vi "SortStates.vi"(0 "object in":refnum<class "StateReverse.lvclass">, 1 "StateTransitions":cluster{"StateTransitions":string[]}[](array[cluster]), 2 "CommentsTransitions":cluster{"StateTransitions":string[]}[](array[cluster]), 3 "StartState":string, 4 "ExitStates":string[](array[string]), 5 "error in (no error)":errorcluster, 8 "StateStrings":string[](array[string]), 9 "RemoveStatesNotInUse(True)":bool=TRUE) -> (14 "object out":refnum<class "StateReverse.lvclass">, 15 "States":T1[](array[typedef]), 19 "error out":errorcluster)   [LabVIEW 2016, in "StateReverse.lvclass"]
uses:
  <resource>/Framework/Providers/Open_GDS/UML/StateReverse_class/StateReverse.lvclass
  <resource>/Framework/Providers/Open_GDS/UML/ReversedEngineering/ReversedEngineering StateMachineStateInfo.ctl
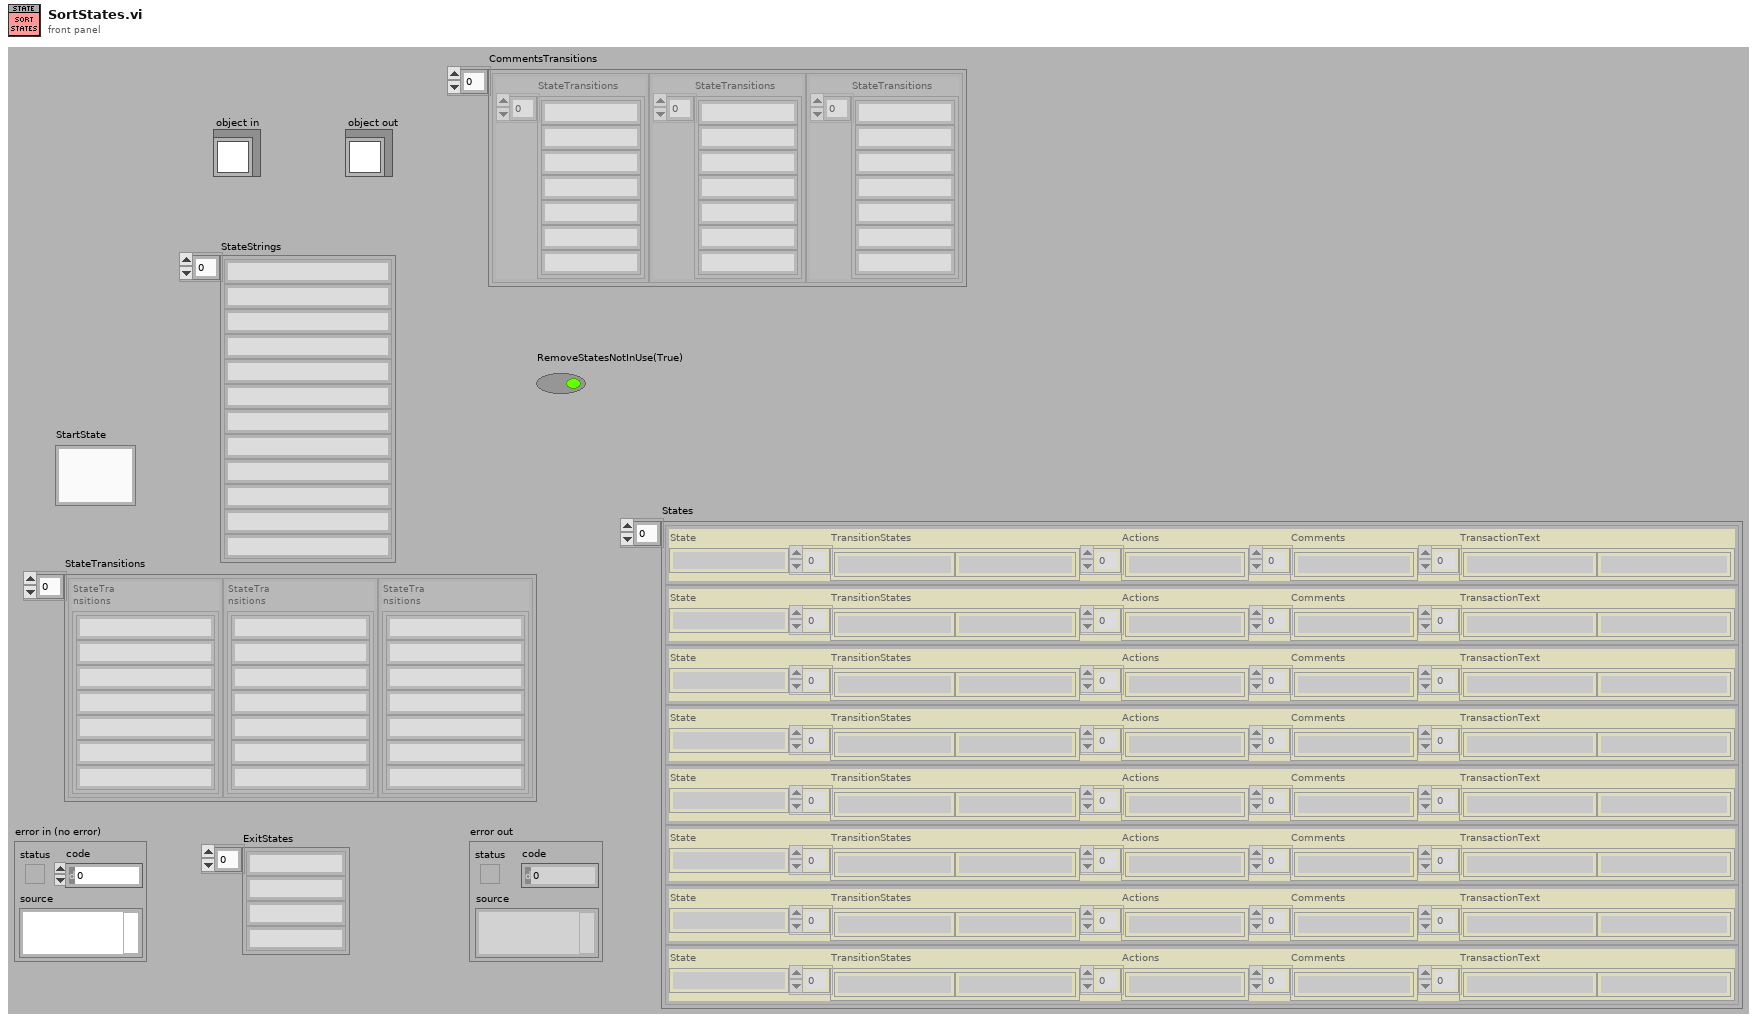
[diagram p1: front panel]
types:
  T1 = typedef "ReversedEngineering StateMachineStateInfo.ctl" = cluster{"State":string, "TransitionStates":string[], "Actions":string[], "Comments":string[], "TransactionText":string[]}
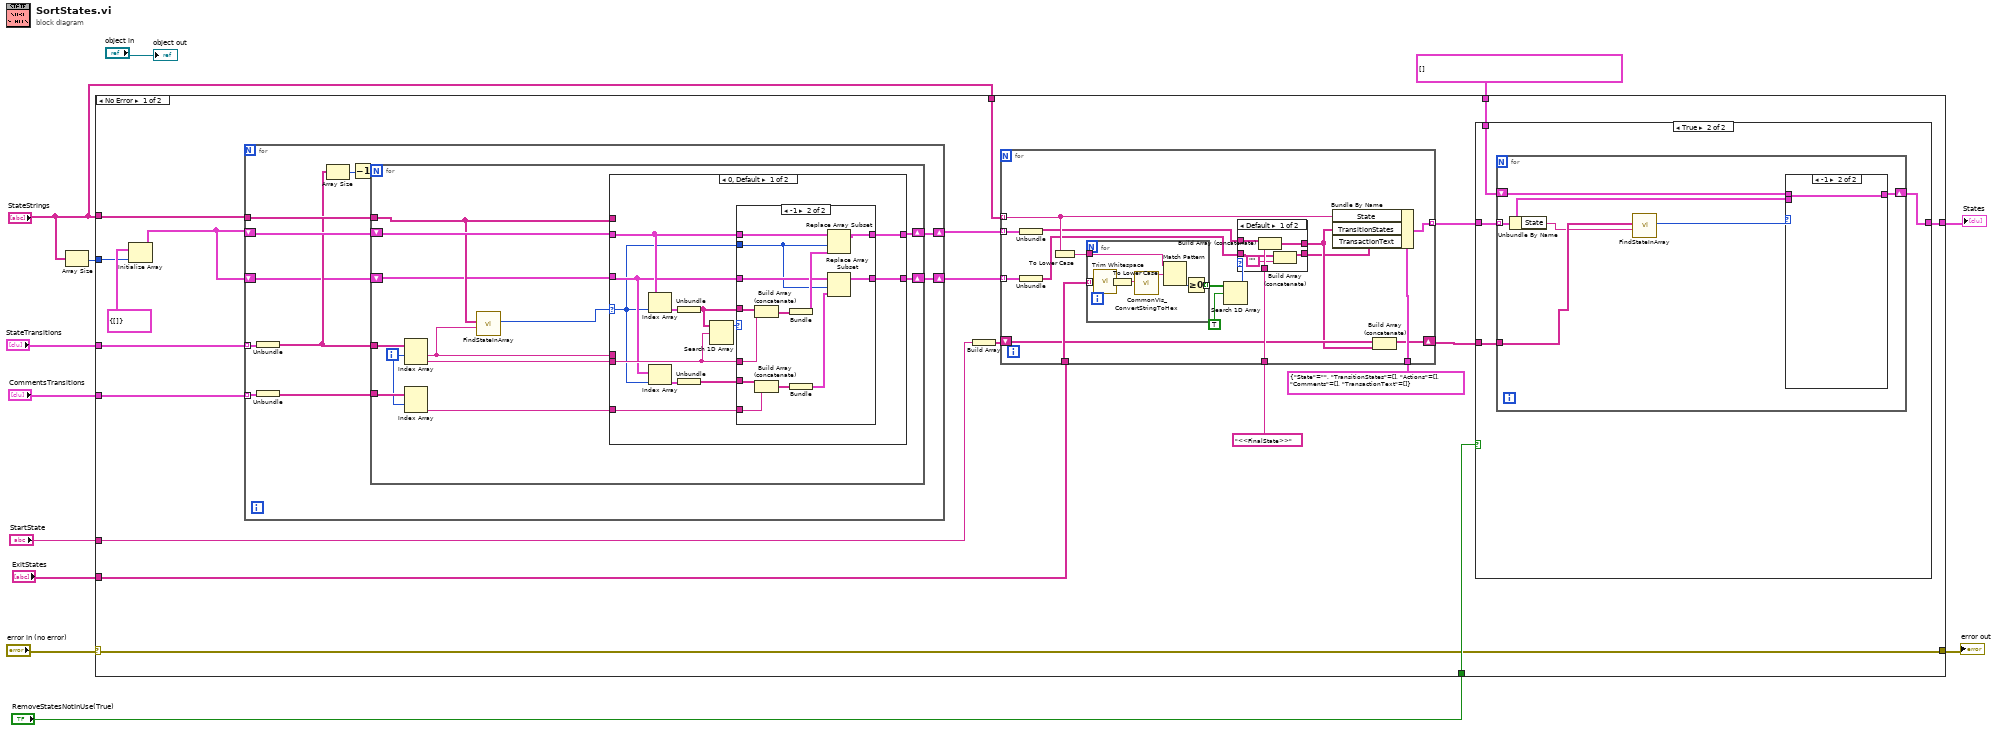
[diagram p0: block diagram]
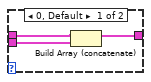
[diagram p3: hidden frame]
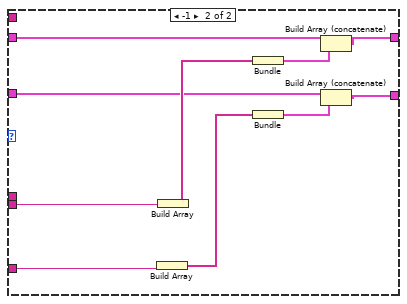
[diagram p6: hidden frame]
diagram:
  n1 = Array Size(array="StateStrings") -> (size(s)=w7:i32)
  n2 = case shown="No Error" "error in (no error)" {
    selector: "error in (no error)" -> [w24 w140]
    tunnel: [w24 w140] -> w11
    tunnel: "StateTransitions" -> [w32 _]
    tunnel: [w22 _] -> w9
    tunnel: "StateStrings" -> [w17 _]
    tunnel: "StateStrings" -> [w29 _]
    tunnel: w7 -> [w27 _]
    tunnel: "ExitStates" -> [w16 _]
    tunnel: "RemoveStatesNotInUse(True)" -> [w25 _]
    tunnel: T1[] [] -> [w20 _]
    tunnel: "StartState" -> [w19 _]
    tunnel: "CommentsTransitions" -> [w14 _]
    frame No Error {
      n3 = Initialize Array(cluster{string[]} {[]}, w27) -> (w15:cluster{string[]}[])
      n4 = for {
        tunnel: w32 -> [w89] mode=indexing
        shift-right: [w87] -> w31
        shift-left: w15 -> [w88]
        tunnel: w17 -> [w90]
        shift-right: [w80] -> w13
        shift-left: w15 -> [w83]
        tunnel: w14 -> [w82] mode=indexing
        n5 = Unbundle(w89) -> ("StateTransitions"=w84:string[])
        n6 = Unbundle(w82) -> ("StateTransitions"=w81:string[])
        n7 = Array Size(array=w84) -> (size(s)=w86:i32)
        n8 = Decrement(x=w86) -> (x-1=w85:i32)
        n9 = for {
          N: w85 -> [_]
          tunnel: w84 -> [w102]
          shift-right: [w100] -> w87
          shift-left: w88 -> [w101]
          tunnel: w90 -> [w98]
          shift-right: [w92] -> w80
          shift-left: w83 -> [w93]
          tunnel: w81 -> [w95]
          i -> [w94]
          n10 = Index Array(array=w102, index #1=w94) -> (element #1=w97:string, element #2=w99:string)  [unwired: 1 in]
          n11 = Index Array(array=w95, index #1=w94) -> (element #2=w91:string)  [unwired: 1 in, 1 out]
          n12 = call <resource>:"FindStateInArray.vi"("TransactionState"=w97, "AllCaseStates"=w98) -> ("index of element"=w96:i32)  [unwired: 7 in, 2 out]
          n13 = case shown="0, Default" w96 {
            selector: w96 -> [w105 _]
            tunnel: w98 -> [_ _]
            tunnel: w97 -> [_ _]
            tunnel: w101 -> [w114 w139]
            tunnel: [w113 w138] -> w100
            tunnel: w99 -> [w110 w136]
            tunnel: w93 -> [w106 w133]
            tunnel: [w108 w132] -> w92
            tunnel: w91 -> [w103 w131]
            frame 0, Default {
              n14 = Index Array(array=w114, index=w105) -> (element=w112:cluster{string[]})
              n15 = Index Array(array=w106, index=w105) -> (element=w107:cluster{string[]})
              n16 = Unbundle(w112) -> (w111:string[])
              n17 = Unbundle(w107) -> (w104:string[])
              n18 = Search 1D Array(1D array=w111, element=w110) -> (index of element=w109:i32)  [unwired: 1 in]
              n19 = case shown="-1" w109 {
                tunnel: w114 -> [w116 w129]
                tunnel: [w116 w128] -> w113
                tunnel: w105 -> [_ w122]
                tunnel: w111 -> [_ w125]
                tunnel: w110 -> [_ w121]
                tunnel: w106 -> [w115 w124]
                tunnel: [w115 w123] -> w108
                tunnel: w104 -> [_ w120]
                tunnel: w103 -> [_ w117]
                frame 0, Default {
                }
                frame -1 {
                  n20 = Build Array (concatenate)(w125, w121) -> (w127:string[])
                  n21 = Build Array (concatenate)(w120, w117) -> (w119:string[])
                  n22 = Bundle(w127) -> (w126:cluster{string[]})  [unwired: 1 in]
                  n23 = Bundle(w119) -> (w118:cluster{string[]})  [unwired: 1 in]
                  n24 = Replace Array Subset(array=w129, new element=w126, index=w122) -> (w128:cluster{string[]}[])
                  n25 = Replace Array Subset(array=w124, new element=w118, index=w122) -> (w123:cluster{string[]}[])
                }
              }
            }
            frame -1 {
              n26 = Build Array(w131) -> (w130:string[])
              n27 = Build Array(w136) -> (w135:string[])
              n28 = Bundle(w135) -> (w137:cluster{string[]})  [unwired: 1 in]
              n29 = Bundle(w130) -> (w134:cluster{string[]})  [unwired: 1 in]
              n30 = Build Array (concatenate)(w139, w137) -> (w138:cluster{string[]}[])
              n31 = Build Array (concatenate)(w133, w134) -> (w132:cluster{string[]}[])
            }
          }
        }
      }
      n32 = Build Array(w19) -> (w18:string[])
      n33 = for {
        tunnel: w31 -> [w64] mode=indexing
        tunnel: T1 {"State"="", "TransitionStates"=[], "Actions"=[], "Comments"=[], "TransactionText"=[]} ("State") -> [w63]
        tunnel: [w62] -> w23 mode=indexing
        tunnel: w29 -> [w58] mode=indexing
        tunnel: w16 -> [w59]
        tunnel: "<<FinalState>>" ("State") -> [w54]
        shift-right: [w52] -> w21
        shift-left: w18 -> [w53]
        tunnel: w13 -> [w50] mode=indexing
        n34 = Unbundle(w64) -> (w55:string[])
        n35 = Unbundle(w50) -> (w49:string[])
        n36 = To Lower Case(string=w58) -> (all lower case string=w60:string)
        n37 = for {
          tunnel: [w79] -> w61 mode=indexing
          tunnel: w60 -> [w78]
          tunnel: w59 -> [w75] mode=indexing
          n38 = call <vilib>:"Trim Whitespace.vi"("string"=w75) -> ("trimmed string"=w73:string)  [unwired: 1 in]
          n39 = To Lower Case(string=w73) -> (all lower case string=w77:string)
          n40 = call <resource>:"CommonVIs_ConvertStringToHex.vi"("inputString"=w77) -> ("outputString"=w76:string)  [unwired: 1 in, 17 out]
          n41 = Match Pattern(string=w78, regular expression=w76) -> (offset past match=w74:i32)  [unwired: 4 out]
          n42 = Greater Or Equal To 0?(x=w74) -> (x >= 0?=w79:bool)
        }
        n43 = Search 1D Array(1D array=w61, element=TRUE) -> (index of element=w56:i32)  [unwired: 1 out]
        n44 = case shown="Default" w56 {
          tunnel: w55 -> [w70 w72]
          tunnel: [w69 w72] -> w51
          tunnel: w54 -> [w68 _]
          tunnel: w49 -> [w66 w71]
          tunnel: [w67 w71] -> w48
          frame Default {
            n45 = Build Array (concatenate)(w70, w68) -> (w69:string[])
            n46 = Build Array (concatenate)(w66, "") -> (w67:string[])
          }
          frame -1 {
          }
        }
        n47 = Bundle By Name(cluster=w63, "State"=w58, "TransitionStates"=w51, "TransactionText"=w48) -> (w62:T1)
        n48 = Build Array (concatenate)(w53, w51) -> (w52:string[])
      }
      n49 = case shown="True" w25 {
        tunnel: w23 -> [w33 w37]
        tunnel: [w33 w34] -> w22
        tunnel: w21 -> [_ w36]
        tunnel: w20 -> [_ w35]
        frame False {
        }
        frame True {
          n50 = for {
            tunnel: w37 -> [w42] mode=indexing
            tunnel: w36 -> [w40]
            shift-right: [w41] -> w34
            shift-left: w35 -> [w43]
            n51 = Unbundle By Name(w42) -> ("State"=w39:string)
            n52 = call <resource>:"FindStateInArray.vi"("TransactionState"=w39, "AllCaseStates"=w40) -> ("index of element"=w38:i32)  [unwired: 7 in, 2 out]
            n53 = case shown="-1" w38 {
              tunnel: w43 -> [w46 w47]
              tunnel: w42 -> [w45 _]
              tunnel: [w44 w47] -> w41
              frame 0, Default {
                n54 = Build Array (concatenate)(w46, w45) -> (w44:T1[])
              }
              frame -1 {
              }
            }
          }
        }
      }
    }
    frame Error {
    }
  }
  "error out" <- w11
  "States" <- w9
  "object out" <- "object in"
